vi "Caller.vi"(0 "Add in":refnum<class "Add.lvclass">, 5 "Sub Panel":refnum<vi>, 7 "Stop":refnum<user-event>, 9 "Class Data":refnum<user-event>, 11 "Error In":errorcluster) -> (4 "Add out":refnum<class "Add.lvclass">, 15 "Error Out":errorcluster)   [LabVIEW 2023, in "Add.lvclass"]
doc: "The VI asynchronously calls the Operation UI method of the addition operation."
uses:
  Add.lvclass
  C:/Users/Ancy.Augustin/Downloads/LVOOPS DVR/LVOOPS DVR/Classes/Arithemtic Operation/Arithemetic Operation.lvclass
  Arithemtic Operation/Arithemetic Operation.lvclass
  Operation UI.vi
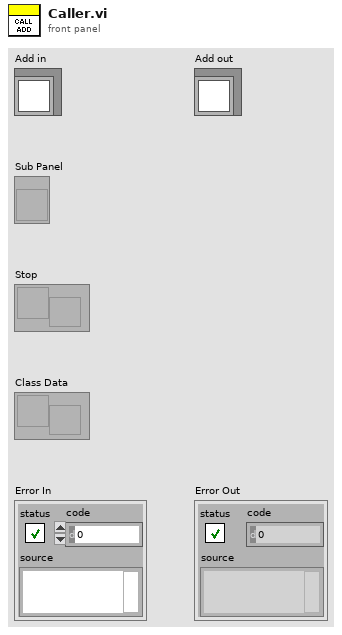
[diagram p1: front panel]
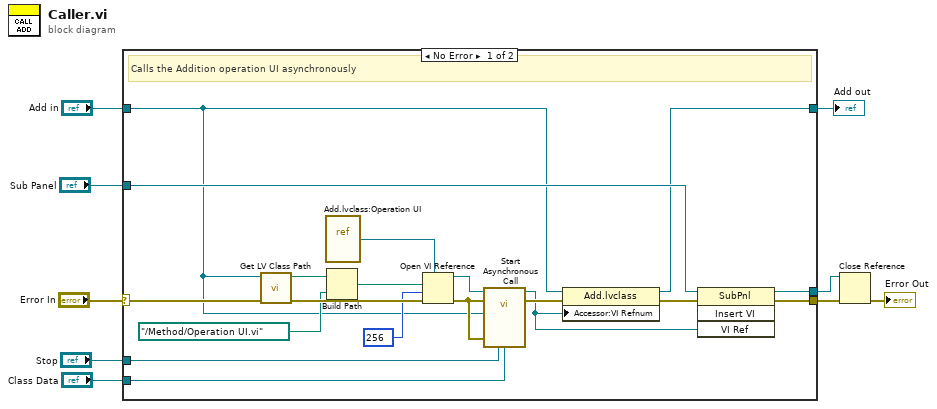
[diagram p0: block diagram]
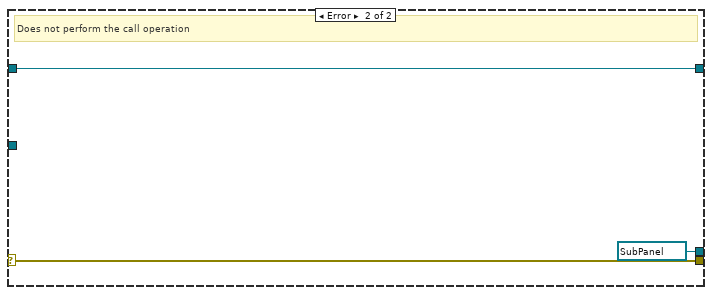
[diagram p2: hidden frame]
diagram:
  n1 = case shown="No Error" "Error In" {
    selector: "Error In" -> [w22 w31]
    tunnel: [w18 w31] -> w8
    tunnel: [w13 w30] -> w6
    tunnel: "Add in" -> [w12 w30]
    tunnel: "Stop" -> [w21 _]
    tunnel: "Class Data" -> [w20 _]
    tunnel: "Sub Panel" -> [w17 _]
    tunnel: [w16 refnum<vi> refnum ("Sub Panel")] -> w1
    frame No Error {
      # "Calls the Addition operation UI asynchronously"
      n2 = call <vilib>:"Get LV Class Path.vi"("error in (no error)"=w22, "object"=w12) -> ("error out"=w28:errorcluster, "class path"=w27:path)  [unwired: 8 in]
      n3 = vi-ref "Add.lvclass:Operation UI.vi"() -> (w11:refnum<vi>)
      n4 = Build Path(base path=w27, name or relative path=path "../Method/Operation UI.vi") -> (appended path=w10:path)
      n5 = Open VI Reference(type specifier VI Refnum (for type only)=w11, vi path=w10, options=256, error in (no error)=w28) -> (vi reference=w23:refnum<vi>, error out=w19:errorcluster)  [unwired: 2 in]
      n6 = call-by-ref "Start Asynchronous Call"(reference=w23, error in=w19, "Add in"=w12, "Error In"=w19, "Stop"=w21, "Class Data"=w20) -> (reference out=w14:refnum<vi>, error out=w25:errorcluster)  [unwired: 9 in, 3 out]
      n7 = property class="Add.lvclass"(reference=w12, error in=w25, "Accessor:VI Refnum"=w14) -> (reference out=w13:refnum<class "Add.lvclass">, error out=w15:errorcluster)
      n8 = invoke class="SubPnl" method="Insert VI"(reference=w17, error in=w15, "VI Ref"=w14) -> (reference out=w16:refnum<vi>, error out=w18:errorcluster)  [unwired: 1 in, 2 out]
    }
    frame Error {
      # "Does not perform the call operation"
    }
  }
  "Add out" <- w6
  n9 = Close Reference(reference=w1, error in (no error)=w8) -> (error out=→"Error Out":errorcluster)
